vi "XML Read Tag Array.vi"(2 "XML content":string[](array[string]), 3 "XML Tag":string) -> (0 "Contents":string[](array[string]), 1 "Tags":string[](array[string]))   [LabVIEW 2015]
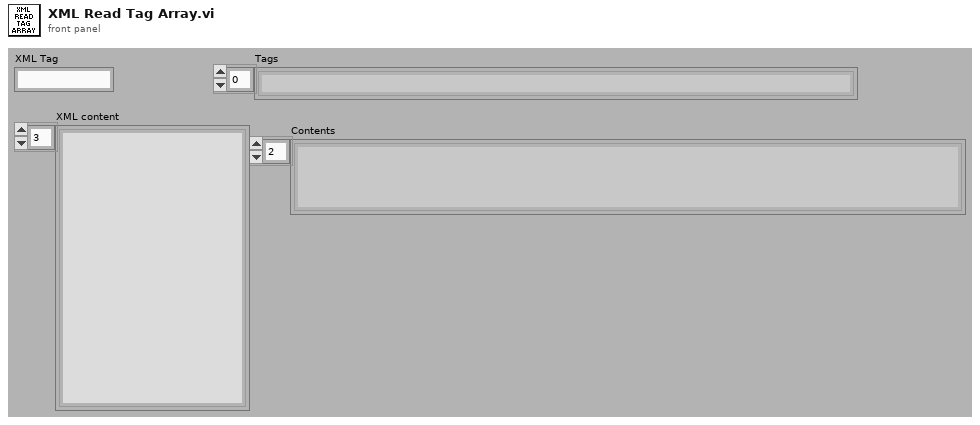
[diagram p1: front panel]
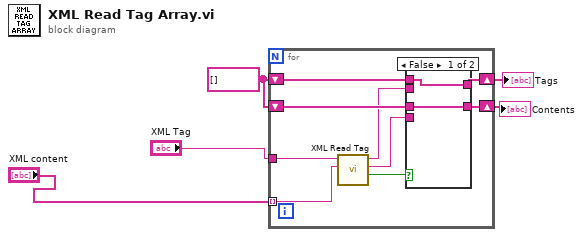
[diagram p0: block diagram]
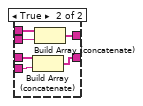
[diagram p2: hidden frame]
diagram:
  w4 = string[] []
  n1 = for {
    tunnel: "XML content" -> [w14] mode=indexing
    shift-right: [w10] -> w2
    shift-left: w4 -> [w11]
    shift-right: [w7] -> w3
    shift-left: w4 -> [w8]
    tunnel: "XML Tag" -> [w6]
    n2 = call "XML Read Tag.vi"("XML"=w14, "XML Tag"=w6) -> ("Found"=w13:bool, "content"=w12:string, "tag parameter"=w9:string)  [unwired: 7 in]
    n3 = case shown="False" w13 {
      tunnel: w12 -> [_ w22]
      tunnel: w11 -> [w15 w21]
      tunnel: [w15 w20] -> w10
      tunnel: w9 -> [_ w19]
      tunnel: w8 -> [w16 w18]
      tunnel: [w16 w17] -> w7
      frame False {
      }
      frame True {
        n4 = Build Array (concatenate)(w21, w22) -> (w20:string[])
        n5 = Build Array (concatenate)(w18, w19) -> (w17:string[])
      }
    }
  }
  "Contents" <- w2
  "Tags" <- w3
